vi "Get Type Name.vi"(11 "Power Supply in":refnum<class "Power Supply.lvclass">) -> (2 "Type Name":string)   [LabVIEW 2020, in "2. Basic Panel Actors.lvlib" / "Power Supply.lvclass"]
doc: "Returns the instrument type name.\n----\nCopyright: MGI 2017\nAuthor: Derek Trepanier"
uses:
  Power Supply.lvclass
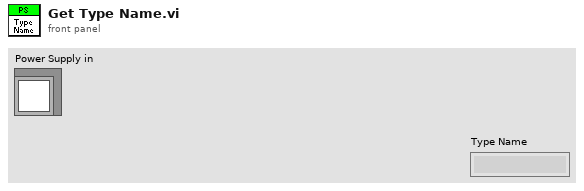
[diagram p1: front panel]
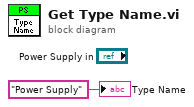
[diagram p0: block diagram]
diagram:
  "Type Name" <- "Power Supply" ("Type Name")
